vi "05_1.vi"() -> ()   [LabVIEW 2018]
panel:
  out "max value":u32
  in  "String":string
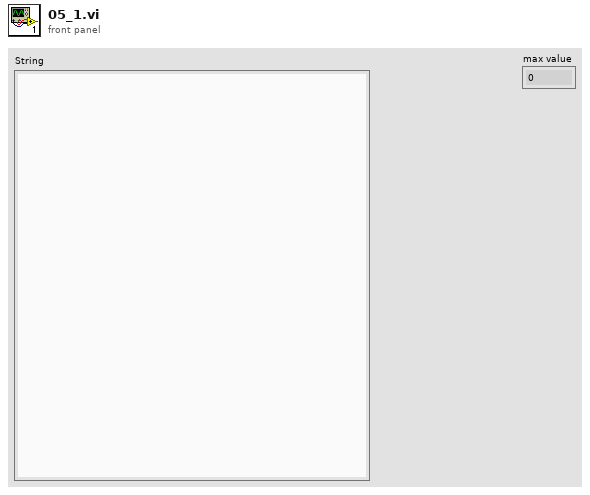
[diagram p1: front panel]
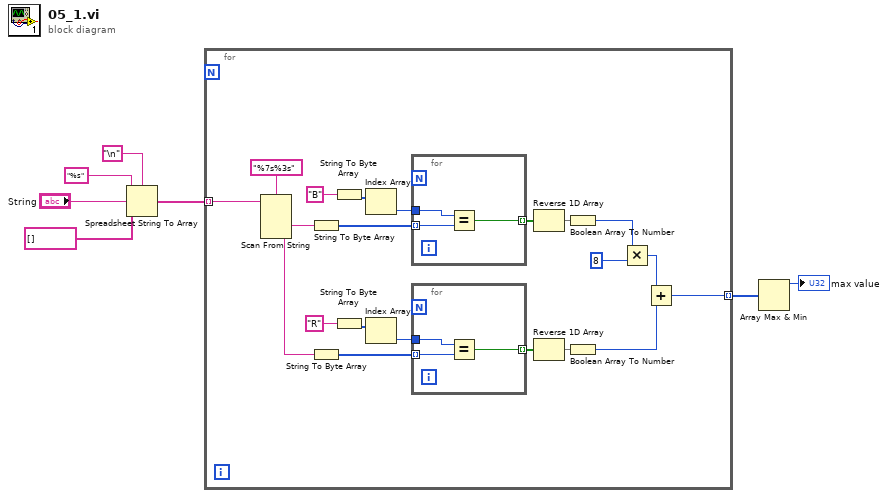
[diagram p0: block diagram]
diagram:
  n1 = Spreadsheet String To Array(delimiter (Tab)="\n", format string="%s", spreadsheet string="String", array type (2D Dbl)=string[] []) -> (array=w3:string[])
  n2 = for {
    tunnel: w3 -> [w28] mode=indexing
    tunnel: [w10] -> w2 mode=indexing
    n3 = Scan From String(format string="%7s%3s", input string=w28) -> (output 1=w26:string, output 2=w15:string)  [unwired: 4 in, 3 out]
    n4 = String To Byte Array(string=w26) -> (unsigned byte array=w25:u8[])
    n5 = String To Byte Array(string=w15) -> (unsigned byte array=w16:u8[])
    n6 = String To Byte Array(string="B") -> (unsigned byte array=w22:u8[])
    n7 = String To Byte Array(string="R") -> (unsigned byte array=w19:u8[])
    n8 = Index Array(array=w22) -> (element=w21:u8)  [unwired: 1 in]
    n9 = Index Array(array=w19) -> (element=w20:u8)  [unwired: 1 in]
    n10 = for {
      tunnel: w25 -> [w34] mode=indexing
      tunnel: [w33] -> w24 mode=indexing
      tunnel: w21 -> [w32]
      n11 = Equal?(x=w32, y=w34) -> (x = y?=w33:bool)
    }
    n12 = for {
      tunnel: w16 -> [w31] mode=indexing
      tunnel: [w30] -> w17 mode=indexing
      tunnel: w20 -> [w29]
      n13 = Equal?(x=w29, y=w31) -> (x = y?=w30:bool)
    }
    n14 = Reverse 1D Array(array=w24) -> (reversed array=w14:bool[])
    n15 = Reverse 1D Array(array=w17) -> (reversed array=w13:bool[])
    n16 = Boolean Array To Number(Boolean array=w14) -> (number=w9:u32)
    n17 = Boolean Array To Number(Boolean array=w13) -> (number=w8:u32)
    n18 = Multiply(x=w9, y=8) -> (x*y=w11:u32)
    n19 = Add(x=w11, y=w8) -> (x+y=w10:u32)
  }
  n20 = Array Max & Min(array=w2) -> (max value=→"max value":u32)  [unwired: 3 out]
